vi "StartVeriStandBundle_Create Reference Locals.vi"(5 "Sequence Context":refnum<k7>) -> (0 "error out":errorcluster)   [LabVIEW 2013, in "MiscHelperVIs.lvlib"]
uses:
  MiscHelperVIs.lvlib
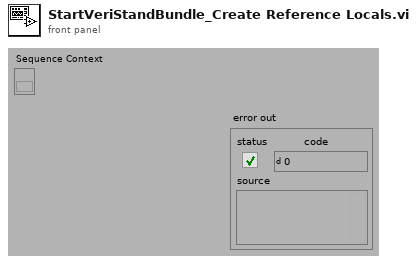
[diagram p1: front panel]
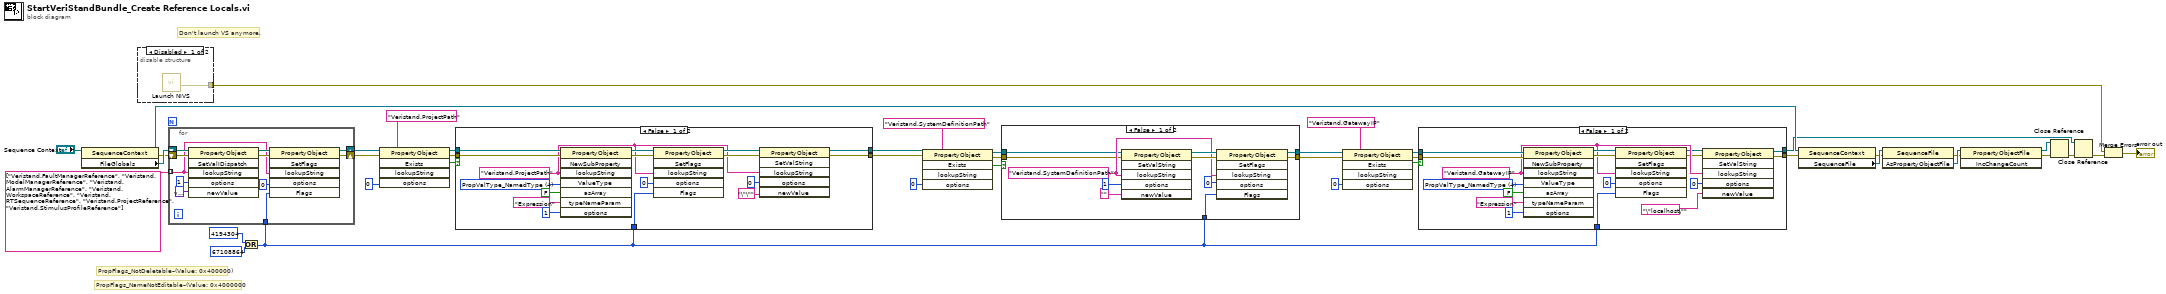
[diagram p0: block diagram]
diagram:
  # "PropFlags_NotDeletable–(Value: 0x400000)"
  # "PropFlags_NameNotEditable–(Value: 0x4000000"
  # "Don't launch VS anymore."
  n1 = property class="SequenceContext"(reference="Sequence Context") -> (reference out=w39:refnum<k7>, error out=w30:errorcluster, "FileGlobals"=w41:refnum<k7>)  [unwired: 1 in]
  n2 = disable-structure shown="Disabled" {
    disable-tunnel: [w42 _] -> w27
    frame Disabled {
      n3 = call "Launch NIVS.vi"() -> ("error out"=w42:errorcluster)  [unwired: 11 in]
    }
    frame Enabled {
    }
  }
  n4 = Or(x=4194304 ("Flags"), y=67108864 ("Flags")) -> (x .or. y?=w20:i32)
  n5 = for {
    shift-right: [w47] -> w26
    shift-left: w41 -> [w53]
    tunnel: string[] ["Veristand.FaultManagerReference", "Veristand.ModelManagerReference", "Veristand.AlarmManagerReference", "Veristand.WorkspaceReference", "Veristand.RTSequenceReference", "Veristand.ProjectReference", "Veristand.StimulusProfileReference"] -> [w43] mode=indexing
    shift-right: [w46] -> w25
    shift-left: w30 -> [w50]
    tunnel: w20 -> [w45]
    n6 = invoke class="PropertyObject" method="SetValIDispatch"(reference=w53, error in=w50, "lookupString"=w43, "options"=1, "newValue"=variant) -> (reference out=w49:refnum<k7>, error out=w48:errorcluster)  [unwired: 1 in, 4 out]
    n7 = invoke class="PropertyObject" method="SetFlags"(reference=w49, error in=w48, "lookupString"=w43, "options"=0, "Flags"=w45) -> (reference out=w47:refnum<k7>, error out=w46:errorcluster)  [unwired: 1 in, 4 out]
  }
  n8 = invoke class="PropertyObject" method="Exists"(reference=w26, error in=w25, "lookupString"="Veristand.ProjectPath", "options"=0) -> (reference out=w2:refnum<k7>, error out=w3:errorcluster, "Exists"=w1:bool)  [unwired: 1 in, 2 out]
  n9 = case shown="False" w1 {
    tunnel: w2 -> [w70 w72]
    tunnel: w3 -> [w69 w71]
    tunnel: [w55 w71] -> w16
    tunnel: [w54 w72] -> w17
    tunnel: w20 -> [w62 _]
    frame False {
      w67 = 4 items=["PropValType_Container", "PropValType_String", "PropValType_Boolean", "PropValType_Number", "PropValType_NamedType", "PropValType_Reference", "PropValType_Array"] ("ValueType")
      w58 = "Veristand.ProjectPath"
      n10 = invoke class="PropertyObject" method="NewSubProperty"(reference=w70, error in=w69, "lookupString"=w58, "ValueType"=w67, "asArray"=FALSE, "typeNameParam"="Expression", "options"=1) -> (reference out=w64:refnum<k7>, error out=w63:errorcluster)  [unwired: 1 in, 6 out]
      n11 = invoke class="PropertyObject" method="SetFlags"(reference=w64, error in=w63, "lookupString"=w58, "options"=0, "Flags"=w62) -> (reference out=w60:refnum<k7>, error out=w59:errorcluster)  [unwired: 1 in, 4 out]
      n12 = invoke class="PropertyObject" method="SetValString"(reference=w60, error in=w59, "lookupString"=w58, "options"=0, "newValue"="\"\"") -> (reference out=w54:refnum<k7>, error out=w55:errorcluster)  [unwired: 1 in, 4 out]
    }
    frame True {
    }
  }
  n13 = invoke class="PropertyObject" method="Exists"(reference=w17, error in=w16, "lookupString"="Veristand.SystemDefinitionPath", "options"=0) -> (reference out=w7:refnum<k7>, error out=w6:errorcluster, "Exists"=w8:bool)  [unwired: 1 in, 2 out]
  n14 = case shown="False" w8 {
    tunnel: w20 -> [w77 _]
    tunnel: [w76 w84] -> w19
    tunnel: [w75 w85] -> w18
    tunnel: w7 -> [w74 w85]
    tunnel: w6 -> [w73 w84]
    frame False {
      w78 = "Veristand.SystemDefinitionPath"
      n15 = invoke class="PropertyObject" method="SetValString"(reference=w74, error in=w73, "lookupString"=w78, "options"=1, "newValue"="") -> (reference out=w80:refnum<k7>, error out=w79:errorcluster)  [unwired: 1 in, 4 out]
      n16 = invoke class="PropertyObject" method="SetFlags"(reference=w80, error in=w79, "lookupString"=w78, "options"=0, "Flags"=w77) -> (reference out=w75:refnum<k7>, error out=w76:errorcluster)  [unwired: 1 in, 4 out]
    }
    frame True {
    }
  }
  n17 = invoke class="PropertyObject" method="Exists"(reference=w18, error in=w19, "lookupString"="Veristand.GatewayIP", "options"=0) -> (reference out=w14:refnum<k7>, error out=w13:errorcluster, "Exists"=w15:bool)  [unwired: 1 in, 2 out]
  n18 = case shown="False" w15 {
    tunnel: w14 -> [w102 w104]
    tunnel: w13 -> [w101 w103]
    tunnel: [w87 w103] -> w21
    tunnel: [w86 w104] -> w22
    tunnel: w20 -> [w94 _]
    frame False {
      w99 = 4 items=["PropValType_Container", "PropValType_String", "PropValType_Boolean", "PropValType_Number", "PropValType_NamedType", "PropValType_Reference", "PropValType_Array"] ("ValueType")
      w90 = "Veristand.GatewayIP"
      n19 = invoke class="PropertyObject" method="NewSubProperty"(reference=w102, error in=w101, "lookupString"=w90, "ValueType"=w99, "asArray"=FALSE, "typeNameParam"="Expression", "options"=1) -> (reference out=w96:refnum<k7>, error out=w95:errorcluster)  [unwired: 1 in, 6 out]
      n20 = invoke class="PropertyObject" method="SetFlags"(reference=w96, error in=w95, "lookupString"=w90, "options"=0, "Flags"=w94) -> (reference out=w89:refnum<k7>, error out=w88:errorcluster)  [unwired: 1 in, 4 out]
      n21 = invoke class="PropertyObject" method="SetValString"(reference=w89, error in=w88, "lookupString"=w90, "options"=0, "newValue"="\"localhost\"") -> (reference out=w86:refnum<k7>, error out=w87:errorcluster)  [unwired: 1 in, 4 out]
    }
    frame True {
    }
  }
  n22 = property class="SequenceContext"(reference=w39, error in=w21) -> (error out=w37:errorcluster, "SequenceFile"=w38:refnum<k7>)  [unwired: 1 out]
  n23 = invoke class="SequenceFile" method="AsPropertyObjectFile"(reference=w38, error in=w37) -> (error out=w35:errorcluster, "AsPropertyObjectFile"=w36:refnum<k7>)  [unwired: 1 in, 1 out]
  n24 = invoke class="PropertyObjectFile" method="IncChangeCount"(reference=w36, error in=w35) -> (reference out=w33:refnum<k7>, error out=w34:errorcluster)  [unwired: 1 in, 1 out]
  n25 = Close Reference(reference=w33, error in (no error)=w34) -> (error out=w32:errorcluster)
  n26 = Close Reference(reference=w22, error in (no error)=w32) -> (error out=w28:errorcluster)
  n27 = Merge Errors(w27, w28) -> (→"error out":errorcluster)
